vi "Clear File Errors.vi"(8 "Error In":errorcluster) -> (0 "Error Out":errorcluster)   [LabVIEW 2013]
doc: "This sub-VI checks for a couple of file I/O errors that can occur through the normal operation of the SVM\nexperiment VI. It clears these errors if they occur so that the user does not worry about errors that are not\nactually critical."
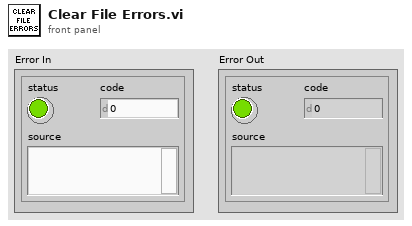
[diagram p1: front panel]
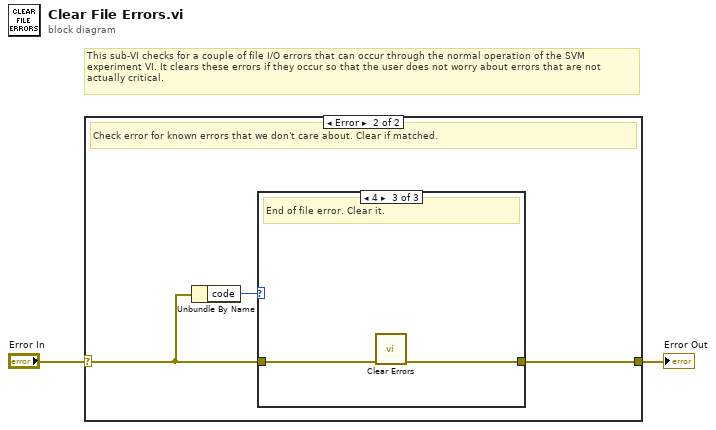
[diagram p0: block diagram]
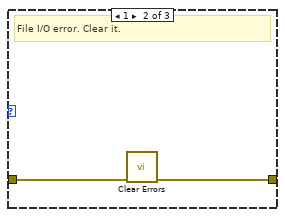
[diagram p4: hidden frame]
diagram:
  # "This sub-VI checks for a couple of file I/O errors that can occur through the normal operation of the SVM\nexperiment VI. It clears these errors if they occur so that the user does not worry about errors that are not\nactually critical."
  n1 = case shown="Error" "Error In" {
    selector: "Error In" -> [w3 w6]
    tunnel: [w3 w4] -> w1
    frame No Error {
      # "No error, so no checks need to be done: pass through and exit"
    }
    frame Error {
      # "Check error for known errors that we don't care about. Clear if matched."
      n2 = Unbundle By Name(w6) -> ("code"=w5:i32)
      n3 = case shown="4" w5 {
        tunnel: w6 -> [w7 w9 w11]
        tunnel: [w7 w8 w10] -> w4
        frame Default {
          # "No match. Pass it through."
        }
        frame 1 {
          # "File I/O error. Clear it."
          n4 = call <vilib>:"Clear Errors.vi"("error in (no error)"=w9) -> ("error out"=w8:errorcluster)  [unwired: 6 in]
        }
        frame 4 {
          # "End of file error. Clear it."
          n5 = call <vilib>:"Clear Errors.vi"("error in (no error)"=w11) -> ("error out"=w10:errorcluster)  [unwired: 6 in]
        }
      }
    }
  }
  "Error Out" <- w1
